vi "Check Trigger Conditions.vi"(6 "Force Trigger?":bool caption="强制触发？", 8 "error in (no error)":errorcluster caption="错误输入（无错误）", 10 "Waveform Data In":waveform(dbl)[](array[waveform]) caption="波形数据输入", 11 "Logging Configuration In":T1 caption="记录配置输入") -> (0 "error out":errorcluster caption="错误输出", 1 "Trigger Conditions Met?":bool caption="触发条件满足？", 2 "Waveform Data Out (copy)":waveform(dbl)[](array[waveform]) caption="图形数据输出（副本）", 3 "Logging Configuration Out":T1 caption="记录配置输出")   [LabVIEW 2013, in "Logging.lvlib"]
doc: "给定记录配置、波形数据和强制触发信息，如果检测到触发将返回真。"
uses:
  Logging.lvlib
  Logging Configuration.ctl
  <vilib>/Analysis/NI_AALPro.lvlib
panel:
  # "（向上滚动可查看记录配置控件）"
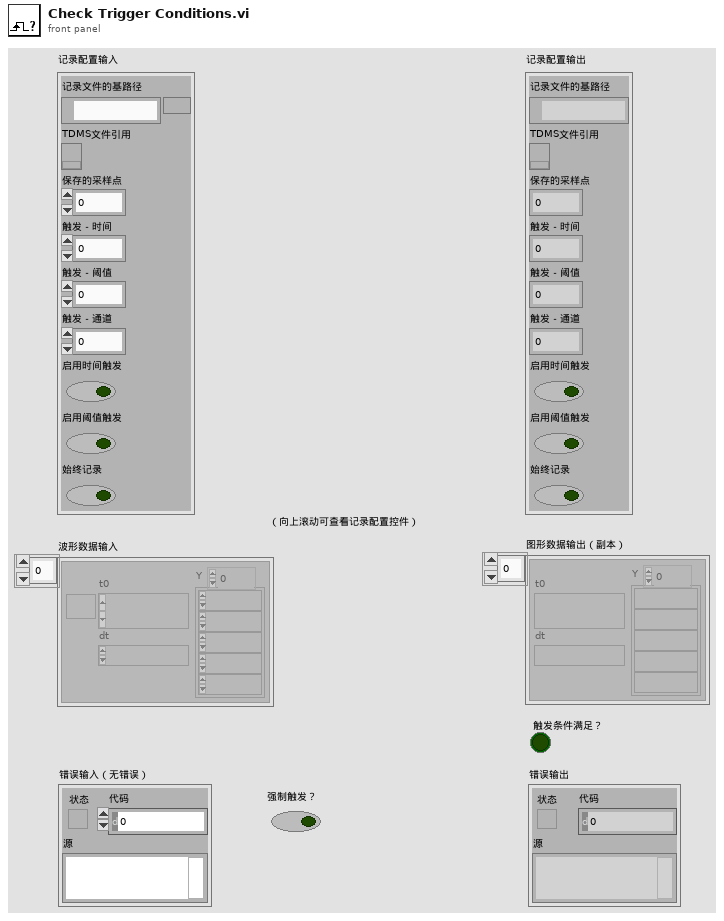
[diagram p1: front panel]
types:
  T1 = typedef "Logging.lvlib/Logging Configuration.ctl" = cluster{"Log File Base Path":path, "TDMS File Reference":refnum<k34>, "Samples to Save":u32, "Trigger - Time":u32, "Trigger - Threshold":dbl, "Trigger - Channel":u32, "Enable Time Trigger":bool, "Enable Threshold Trigger":bool, "Always Log":bool}
  T2 = typedef "LVDateTimeRec.ctl" = cluster{"fractional second":dbl, "second":i32, "minute":i32, "hour":i32, "day of month":i32, "month":i32, "year":i32, "day of week":i32, "day of year":i32, "DST":i32}
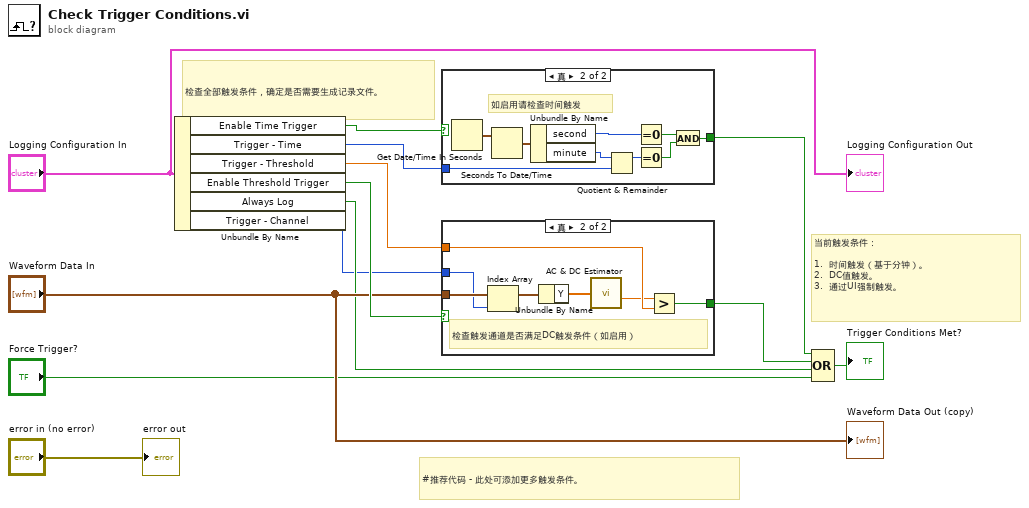
[diagram p0: block diagram]
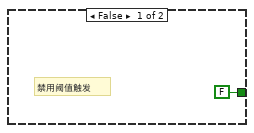
[diagram p2: hidden frame]
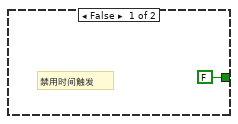
[diagram p3: hidden frame]
diagram:
  # "检查全部触发条件，确定是否需要生成记录文件。"
  # "当前触发条件：\n\n1.  时间触发（基于分钟）。\n2.  DC值触发。\n3.  通过UI强制触发。"
  # "#推荐代码 - 此处可添加更多触发条件。"
  n1 = Unbundle By Name("Logging Configuration In") -> ("Enable Time Trigger"=w8:bool, "Trigger - Time"=w9:u32, "Trigger - Threshold"=w10:dbl, "Enable Threshold Trigger"=w7:bool, "Always Log"=w4:bool, "Trigger - Channel"=w1:u32)
  n2 = case shown="真" w8 {
    tunnel: [FALSE w16] -> w11
    tunnel: w9 -> [_ w15]
    frame False {
      # "禁用时间触发"
    }
    frame True {
      # "如启用请检查时间触发"
      n3 = Get Date/Time In Seconds() -> (seconds since 1Jan1904=w20:timestamp)
      n4 = Seconds To Date/Time(time stamp (now)=w20) -> (date time rec=w23:T2)  [unwired: 1 out]
      n5 = Unbundle By Name(w23) -> ("second"=w22:i32, "minute"=w19:i32)
      n6 = Quotient & Remainder(x=w19, y=w15) -> (x-y*floor(x/y)=w18:u32)  [unwired: 1 out]
      n7 = Equal To 0?(x=w22) -> (x = 0?=w21:bool)
      n8 = Equal To 0?(x=w18) -> (x = 0?=w17:bool)
      n9 = And(x=w21, y=w17) -> (x .and. y?=w16:bool)
    }
  }
  n10 = case shown="真" w7 {
    tunnel: "Waveform Data In" -> [_ w27]
    tunnel: [FALSE w28] -> w13
    tunnel: w10 -> [_ w31]
    tunnel: w1 -> [_ w25]
    frame False {
      # "禁用阈值触发"
    }
    frame True {
      # "检查触发通道是否满足DC触发条件（如启用）"
      n11 = Index Array(array=w27, index=w25) -> (element=w26:waveform(dbl))
      n12 = Unbundle By Name(w26) -> ("Y"=w30:dbl[])
      n13 = call <vilib>:"AC & DC Estimator.vi"("Signal (V)"=w30) -> ("DC estimate (V)"=w29:dbl)  [unwired: 1 out]
      n14 = Greater?(x=w29, y=w31) -> (0:w28:bool)
    }
  }
  n15 = Compound Arithmetic op=OR(w11, w13, w4, "Force Trigger?") -> (→"Trigger Conditions Met?":bool)
  "error out" <- "error in (no error)"
  "Waveform Data Out (copy)" <- "Waveform Data In"
  "Logging Configuration Out" <- "Logging Configuration In"
